vi "Execute.vi"(6 "commandTimeout":i32=-1, 7 "CommandType":i32(ring)=-1 items=["Text"=1, "StoredProcedure"=4, "TableDirect"=512], 8 "error in (no error)":errorcluster, 9 "DynamicParameters":refnum<class "DynamicParameters.lvclass">, 10 "sql":string, 11 "ADOMapper in":refnum<class "ADOMapper.lvclass">) -> (0 "error out":errorcluster, 2 "affectedRows":i32, 3 "ADOMapper out":refnum<class "ADOMapper.lvclass">)   [LabVIEW 2020, in "ORM_ADONet.lvlib" / "ADOMapper.lvclass"]
uses:
  ADOMapper.lvclass
  C:/Program Files/National Instruments/LabVIEW 2020/vi.lib/Viviota/shared/ORM.lvlibp/ORM/SqlMapper/SqlMapper.lvclass
  <vilib>/Viviota/shared/ORM.lvlibp/ORM/DynamicParameters/DynamicParameters.lvclass
  <vilib>/Viviota/shared/ORM_DBC_dotNet.lvlibp/dbcDotNet/ORM_DBC_dotNet.lvclass
  C:/Program Files/National Instruments/LabVIEW 2020/vi.lib/Viviota/shared/ORM.lvlibp/ORM/DbConnection/DbConnection.lvclass
  System.Data
  <vilib>/Viviota/shared/ORM.lvlibp/ORM/SqlMapper/Read DbConnection.vi
  <vilib>/Viviota/shared/ORM.lvlibp/ORM/DbConnection/Read ExecuteScalar.vi
  <vilib>/Viviota/shared/ORM.lvlibp/ORM/DbConnection/Write ExecuteScalar.vi
  <vilib>/Viviota/shared/ORM_DBC_dotNet.lvlibp/dbcDotNet/Read transaction.vi
  <vilib>/Viviota/shared/ORM.lvlibp/ORM/SqlMapper/Write DbConnection.vi
  <vilib>/Viviota/shared/ORM.lvlibp/ORM/DbConnection/DbConnection.lvclass
  <userlib>/_OpenG.lib/error/error.llb/openg_error.lvlib
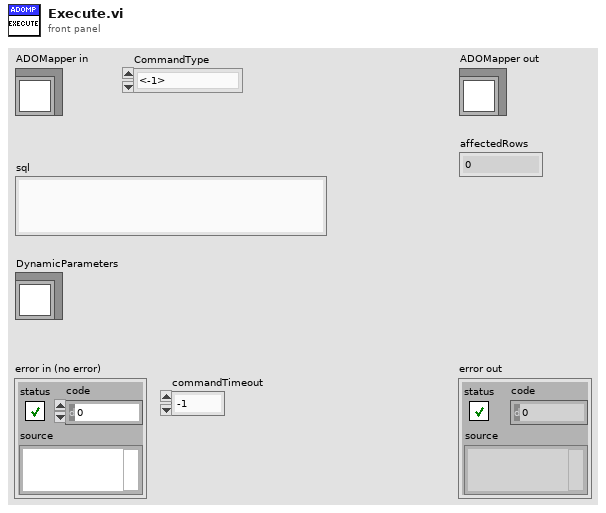
[diagram p1: front panel]
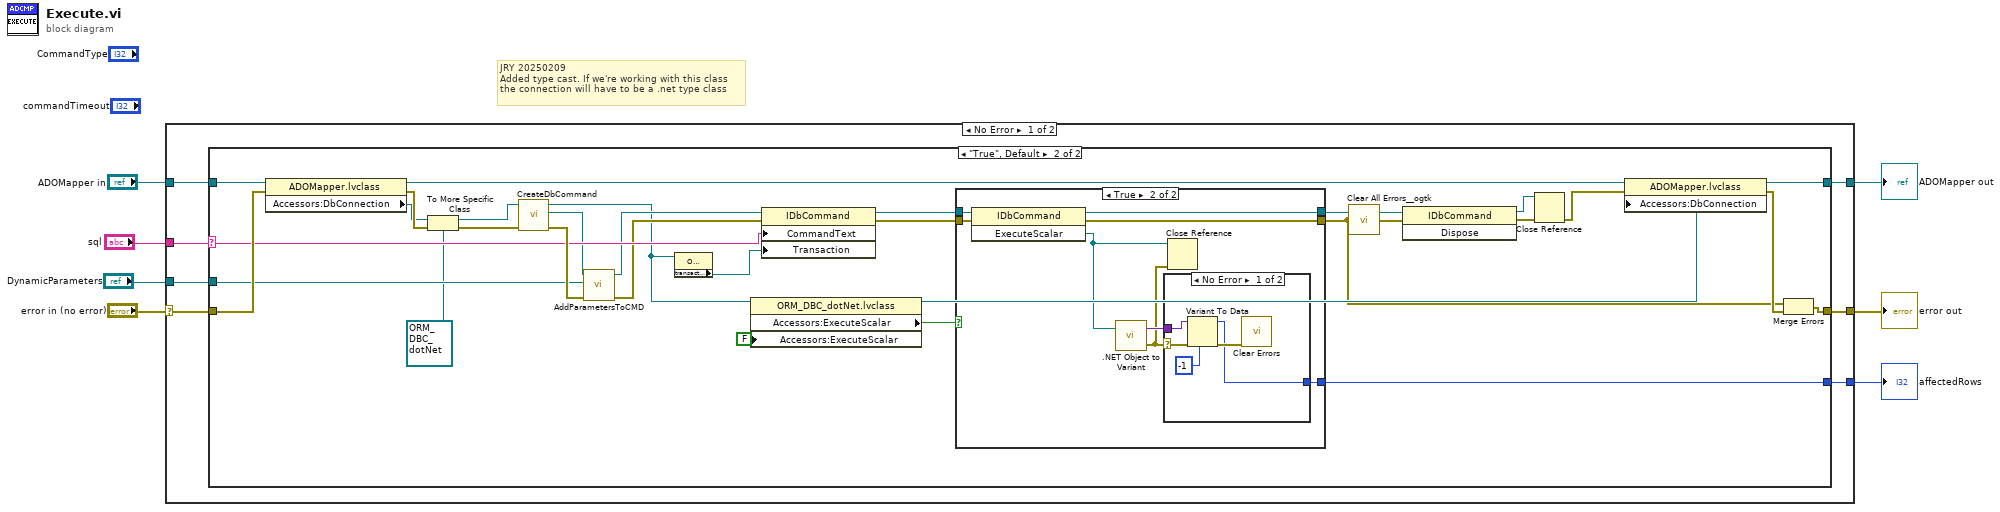
[diagram p0: block diagram]
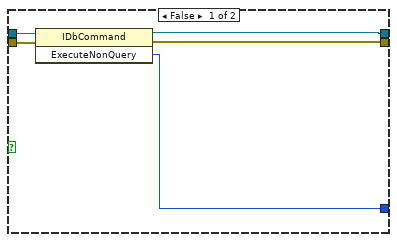
[diagram p3: hidden frame]
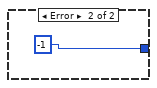
[diagram p4: hidden frame]
diagram:
  # "JRY 20250209\nAdded type cast. If we're working with this class\nthe connection will have to be a .net type class"
  n1 = case shown="No Error" "error in (no error)" {
    selector: "error in (no error)" -> [w12 w68]
    tunnel: "ADOMapper in" -> [w14 w67]
    tunnel: [w13 w67] -> w6
    tunnel: "sql" -> [w11 _]
    tunnel: [w10 _] -> w3
    tunnel: [w9 w68] -> w2
    tunnel: "DynamicParameters" -> [w8 _]
    frame No Error {
      n2 = case shown="\"True\", Default" w11 {
        selector: w11 -> [_ w42]
        tunnel: w14 -> [w16 w47]
        tunnel: [w16 w29] -> w13
        tunnel: w12 -> [w15 w45]
        tunnel: [_ w32] -> w10
        tunnel: [w15 w22] -> w9
        tunnel: w8 -> [_ w34]
        frame "" {
        }
        frame "True", Default {
          n3 = property class="ADOMapper.lvclass"(reference=w47, error in=w45) -> (reference out=w46:refnum<class "ADOMapper.lvclass">, error out=w44:errorcluster, "Accessors:DbConnection"=w19:refnum<class "DbConnection.lvclass">)
          n4 = To More Specific Class(target class=refnum<class "ORM_DBC_dotNet.lvclass"> refnum ("ORM_DBC_dotNet.lvlibp:ORM_DBC_dotNet.lvclass"), reference=w19, error in=w44) -> (specific class reference=w18:refnum<class "ORM_DBC_dotNet.lvclass">, error out=w20:errorcluster)
          n5 = call <vilib>:"CreateDbCommand.vi"("error in (no error)"=w20, "DbConnection in"=w18) -> ("error out"=w43:errorcluster, "CreateCommand"=w35:refnum<k24>, "DbConnection out"=w26:refnum<class "ORM_DBC_dotNet.lvclass">)  [unwired: 7 in]
          n6 = call "AddParametersToCMD.vi"("error in (no error)"=w43, "DynamicParameters in"=w34, "CreateCommand"=w35) -> ("error out"=w40:errorcluster, "CreateCommand Out"=w33:refnum<k24>)  [unwired: 7 in]
          n7 = property class="ORM_DBC_dotNet.lvclass"(reference=w26) -> ("transaction"=w25:refnum<k24>)  [unwired: 1 in, 2 out]
          n8 = property class="ORM_DBC_dotNet.lvclass"(reference=w26, "Accessors:ExecuteScalar"=FALSE ("ExecuteScalar")) -> (reference out=w24:refnum<class "ORM_DBC_dotNet.lvclass">, "Accessors:ExecuteScalar"=w31:bool)  [unwired: 1 in, 1 out]
          n9 = property class="IDbCommand"(reference=w33, error in=w40, "CommandText"=w42, "Transaction"=w25) -> (reference out=w41:refnum<k24>, error out=w39:errorcluster)
          n10 = case shown="True" w31 {
            tunnel: w41 -> [w51 w60]
            tunnel: w39 -> [w52 w59]
            tunnel: [w49 w58] -> w21
            tunnel: [w50 w57] -> w38
            tunnel: [w48 w55] -> w32
            frame False {
              n11 = invoke class="IDbCommand" method="ExecuteNonQuery"(reference=w51, error in=w52) -> (reference out=w50:refnum<k24>, error out=w49:errorcluster, "ExecuteNonQuery"=w48:i32)  [unwired: 1 in]
            }
            frame True {
              n12 = invoke class="IDbCommand" method="ExecuteScalar"(reference=w60, error in=w59) -> (reference out=w57:refnum<k24>, error out=w58:errorcluster, "ExecuteScalar"=w54:refnum<k24>)  [unwired: 1 in]
              n13 = call <vilib>:".NET Object to Variant.vi"(".NET object"=w54) -> ("error out"=w53:errorcluster, "variant"=w56:variant)  [unwired: 1 in]
              n14 = case shown="No Error" w53 {
                selector: w53 -> [w65 _]
                tunnel: w56 -> [w64 _]
                tunnel: [w61 -1] -> w55
                frame No Error {
                  n15 = Variant To Data(error in=w65, type=-1, Variant=w64) -> (data=w61:i32, error out=w62:errorcluster)
                  n16 = call <vilib>:"Clear Errors.vi"("error in (no error)"=w62) -> ()  [unwired: 5 in, 2 out]
                }
                frame Error {
                }
              }
              n17 = Close Reference(reference=w54, error in (no error)=w53) -> ()  [unwired: 1 out]
            }
          }
          n18 = call <userlib>:"Clear All Errors__ogtk.vi"("Error In"=w21) -> ("Error Out"=w23:errorcluster)  [unwired: 3 in]
          n19 = invoke class="IDbCommand" method="Dispose"(reference=w38, error in=w23) -> (reference out=w36:refnum<k24>, error out=w37:errorcluster)  [unwired: 1 in, 1 out]
          n20 = Close Reference(reference=w36, error in (no error)=w37) -> (error out=w28:errorcluster)
          n21 = property class="ADOMapper.lvclass"(reference=w46, error in=w28, "Accessors:DbConnection"=w24) -> (reference out=w29:refnum<class "ADOMapper.lvclass">, error out=w27:errorcluster)
          n22 = Merge Errors(w21, w27) -> (w22:errorcluster)
        }
      }
    }
    frame Error {
    }
  }
  "error out" <- w2
  "ADOMapper out" <- w6
  "affectedRows" <- w3
